vi "Build-timeline.vi"(8 "error in (no error)":errorcluster, 10 "Temp-timeline in":T1, 11 "Attribute in":refnum<class "MarkSpeed.lvclass">) -> (0 "error out":errorcluster, 2 "Temp-timeline":T1, 3 "Attribute out":refnum<class "MarkSpeed.lvclass">)   [LabVIEW 2013, in "HardwareCharacterization.lvlib" / "MarkSpeed.lvclass"]
uses:
  MarkSpeed.lvclass
  ScanParser/Path-buffer.ctl
  ScanParser/Point-buffer.ctl
  Element-XML/Elements.ctl
  ScanParser/Property-buffer.ctl
  ScanParser/Units.ctl
  ScanParser/Speed.ctl
  Speed/Speed.lvclass/Speed.ctl
  Speed/Read Components.vi
  Speed/Read Speed.vi
  Speed/Read Bits per period.vi
  Speed/Read Update period.vi
  ScanParser/HC-ScanParser.lvclass
  Element-XML/Element-XML.lvclass
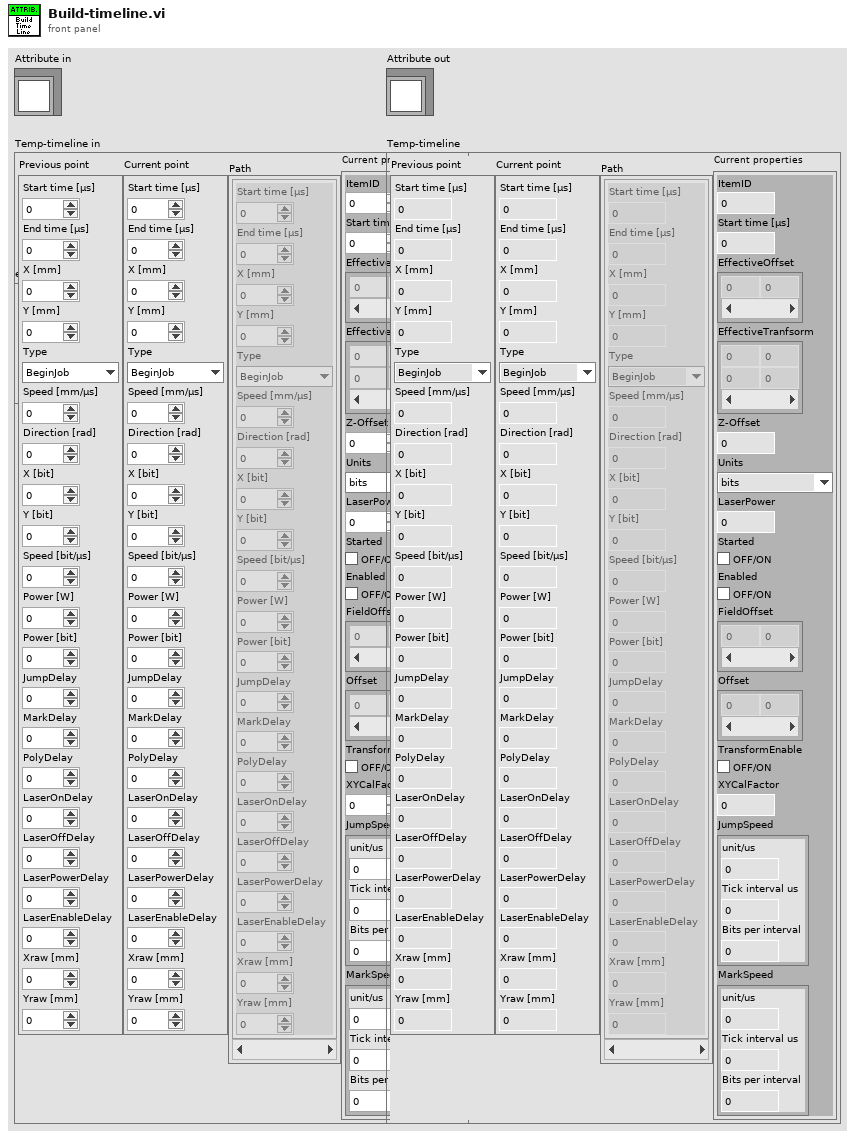
[diagram p1: front panel]
types:
  T1 = typedef "HardwareCharacterization.lvlib/HC-ScanParser.lvclass/Path-buffer.ctl" = cluster{"Previous point":T2, "Current point":T2, "Path":T2[], "Current properties":T4}
  T2 = typedef "HardwareCharacterization.lvlib/HC-ScanParser.lvclass/Point-buffer.ctl" = cluster{"Start time [µs]":i64, "End time [µs]":i64, "X [mm]":dbl, "Y [mm]":dbl, "Type":T3, "Speed [mm/µs]":dbl, "Direction [rad]":dbl, "X [bit]":i16, "Y [bit]":i16, "Speed [bit/µs]":dbl, "Power [W]":dbl, "Power [bit]":u8, "JumpDelay":i64, "MarkDelay":i64, "PolyDelay":i64, "LaserOnDelay":i64, "LaserOffDelay":i64, "LaserPowerDelay":i64, "LaserEnableDelay":i64, "Xraw [mm]":dbl, "Yraw [mm]":dbl}
  T3 = typedef "HardwareCharacterization.lvlib/Element-XML.lvclass/Elements.ctl" = enum16{"BeginJob", "WriteDigital", "WriteAnalog", "Set", "ApplicationEvent", "JumpAbs", "MarkAbs", "JumpRel", "MarkRel", "LongDelay", "EndJob"}
  T4 = typedef "HardwareCharacterization.lvlib/HC-ScanParser.lvclass/Property-buffer.ctl" = cluster{"ItemID":u32, "Start time":i64, "EffectiveOffset":dbl[], "EffectiveTranfsorm":dbl[][], "Z-Offset":sgl, "Units":T5, "LaserPower":u8, "Started":bool, "Enabled":bool, "FieldOffset":dbl[], "Offset":dbl[], "TransformEnable":bool, "XYCalFactor":dbl, "JumpSpeed":T6, "MarkSpeed":T6}
  T5 = typedef "HardwareCharacterization.lvlib/HC-ScanParser.lvclass/Units.ctl" = enum16{"bits", "mm", "inch", "mils"}
  T6 = typedef "HardwareCharacterization.lvlib/HC-ScanParser.lvclass/Speed.ctl" = cluster{"unit/us":dbl, "Tick interval us":u16, "Bits per interval":u16}
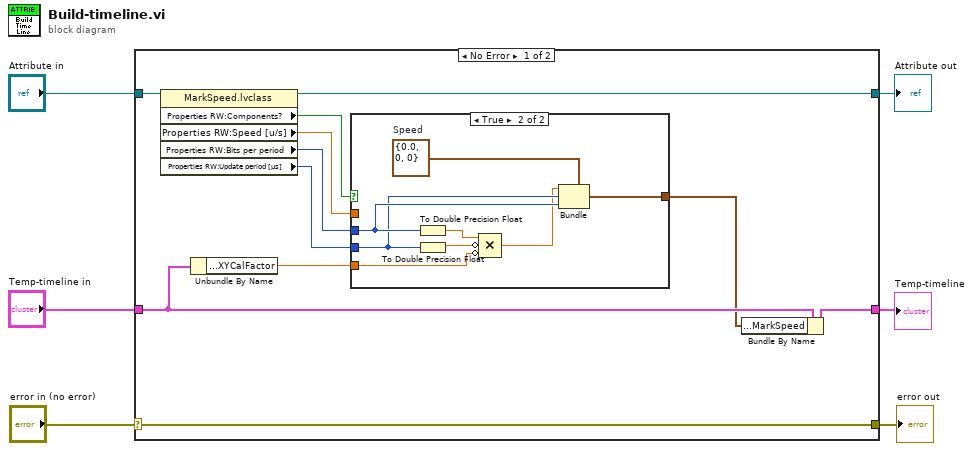
[diagram p0: block diagram]
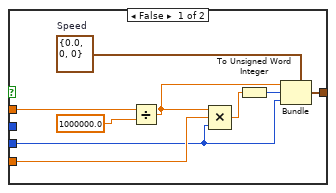
[diagram p2: hidden frame]
diagram:
  n1 = case shown="No Error" "error in (no error)" {
    selector: "error in (no error)" -> [w11 w37]
    tunnel: [w11 w37] -> w5
    tunnel: [w16 w36] -> w3
    tunnel: "Attribute in" -> [w17 w36]
    tunnel: "Temp-timeline in" -> [w9 w35]
    tunnel: [w8 w35] -> w1
    frame No Error {
      n2 = property class="MarkSpeed.lvclass"(reference=w17) -> (reference out=w16:refnum<class "MarkSpeed.lvclass">, "Properties RW:Components?"=w15:bool, "Properties RW:Speed [u/s]"=w14:dbl, "Properties RW:Bits per period"=w13:u16, "Properties RW:Update period [µs]"=w12:u16)  [unwired: 1 in, 1 out]
      n3 = Unbundle By Name(w9) -> ("Current properties.XYCalFactor"=w10:dbl)
      n4 = case shown="True" w15 {
        tunnel: w14 -> [w25 _]
        tunnel: w13 -> [_ w31]
        tunnel: w12 -> [w19 w30]
        tunnel: w10 -> [w20 w28]
        tunnel: [w18 w27] -> w7
        frame False {
          w24 = T6 {"unit/us"=0.0, "Tick interval us"=0, "Bits per interval"=0}  # Speed
          n5 = Divide(x=w25, y=1000000.0) -> (x/y=w21:dbl)
          n6 = Compound Arithmetic op=MULTIPLY(w21, w20, w19) -> (w23:dbl)
          n7 = To Unsigned Word Integer(number=w23) -> (unsigned 16bit integer=w22:u16)
          n8 = Bundle(cluster=w24, "unit/us"=w21, "Tick interval us"=w22, "Bits per interval"=w19) -> (w18:T6)
        }
        frame True {
          w32 = T6 {"unit/us"=0.0, "Tick interval us"=0, "Bits per interval"=0}  # Speed
          n9 = To Double Precision Float(number=w31) -> (double precision float=w33:dbl)
          n10 = To Double Precision Float(number=w30) -> (double precision float=w34:dbl)
          n11 = Compound Arithmetic op=MULTIPLY(w33, invert w34, invert w28) -> (w29:dbl)
          n12 = Bundle(cluster=w32, "unit/us"=w29, "Tick interval us"=w30, "Bits per interval"=w31) -> (w27:T6)
        }
      }
      n13 = Bundle By Name(cluster=w9, "Current properties.MarkSpeed"=w7) -> (w8:T1)
    }
    frame Error {
    }
  }
  "error out" <- w5
  "Attribute out" <- w3
  "Temp-timeline" <- w1
